vi "Class to Variant.vi"(8 "error in (no error)":errorcluster, 10 "Data in":variant, 11 "UTF Node in":refnum<class "UTF Node.lvclass">) -> (0 "error out":errorcluster, 1 "Serialized Object Name":string, 2 "Data Out":variant, 3 "UTF Node out":refnum<class "UTF Node.lvclass">)   [LabVIEW 2014, in "UTF Node.lvclass"]
uses:
  UTF Node.lvclass
  Shared/Controls/Run UTF - STYP.ctl
  UTF Node.lvclass/UTF Node.ctl
  Classes/Build Job/Build Job.lvclass
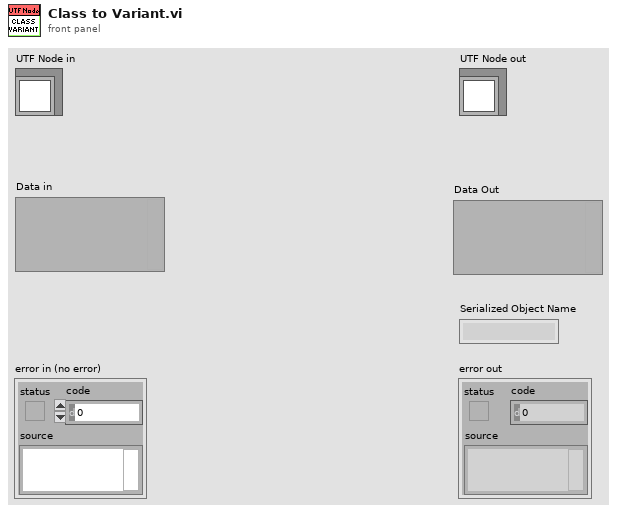
[diagram p1: front panel]
types:
  T1 = typedef "Run UTF - STYP.ctl" = cluster{"Project Path":string}
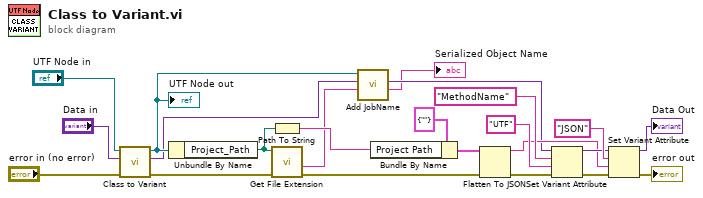
[diagram p0: block diagram]
diagram:
  n1 = call-parent "Class to Variant.vi"("error in (no error)"="error in (no error)", "Data in"="Data in", "Build Job in"="UTF Node in") -> ("error out"=w7:errorcluster, "Data Out"=w3:variant, "Build Job out"=w4:refnum<class "UTF Node.lvclass">)  [unwired: 5 in, 1 out]
  "UTF Node out" <- w4
  n2 = Unbundle By Name(w4) -> ("Project_Path"=w5:path)
  n3 = Path To String(path=w5) -> (string=w19:string)
  n4 = call <vilib>:"Get File Extension.vi"("error in (no error)"=w7, "file"=w5) -> ("error out"=w6:errorcluster, "filename without extension"=w8:string)  [unwired: 6 in, 2 out]
  n5 = call "Add JobName.vi"("Job Target"=w8, "Data in"=w3, "Build Job in"=w4) -> ("Job Name"=→"Serialized Object Name":string, "Data Out"=w2:variant)  [unwired: 7 in]
  n6 = Bundle By Name(cluster=T1 {"Project Path"=""} ("Run UTF"), "Project Path"=w19) -> (w18:T1)
  n7 = Flatten To JSON(anything=w18, error in (no error)=w6) -> (JSON string=w11:string, 11:w10:errorcluster)  [unwired: 1 in]
  n8 = Set Variant Attribute(Variant=w2, name="MethodName", value="UTF", error in=w10) -> (Variant out=w15:variant, error out=w17:errorcluster)  [unwired: 1 out]
  n9 = Set Variant Attribute(Variant=w15, name="JSON" ("Name"), value=w11, error in=w17) -> (Variant out=→"Data Out":variant, error out=→"error out":errorcluster)  [unwired: 1 out]
